vi "Test MFC ESF.vi"() -> ()   [LabVIEW 2015, in "Alicat Device.lvclass"]
uses:
  Alicat Device.lvclass
  Reusable/Session APIs/File Access/Config Data/Config Session.ctl
  Reusable/Session APIs/File Access/Config Data/Config Data.lvclass
  Reusable/Session APIs/Serial/Serial Session.lvclass
  <userlib>/_Session Fwk/Typedefs/Session Handle.ctl
  <userlib>/_Session Fwk/Session - Root.lvclass
  Reusable/Session Log/System Log.lvclass
  Reusable/Session Log/System Log.lvclass/System Log.ctl
  Reusable/Session APIs/File Access/Config Data/Config Data.lvclass/Config Data.ctl
  Reusable/Session APIs/Text Communication/Text Device Session.lvclass/Text Device Session.ctl
  Configurable Device/Configurable Device.lvclass/Configurable Device.ctl
  Alicat Device.lvclass/Alicat Device.ctl
  Data/M/M data.lvclass
  Data/Alicat Data.lvclass
  Data/M/M data.lvclass/M data.ctl
  Reusable/Session APIs/Text Communication/Write hSysLog.vi
  Configurable Device/Write Handle.vi
  Accessors/Write ID.vi
  Accessors/Write Session Handle.vi
  Data/M/Accessors/Read P.vi
  Data/M/Accessors/Read T.vi
  Reusable/Session APIs/File Access/Config Data/Accessors/Write Cfg Path.vi
  Reusable/Session Log/Accessors/Write Main Path.vi
  Reusable/Data/Read measTime.vi
panel:
  out "Numeric":u32
  out "Accessors:Data":sgl[][](array[numeric])
  out "Array 3":errorcluster[](array[cluster])
  out "Array 2":errorcluster[](array[cluster])
  in  "Stop":bool
  in  "Path":path=path "c:/aop/aop.ini"
  in  "Main Path":path=path "c:/aop/logs"
  in  "Array":string[](array[string])=["CRDS_Purge", "CRDS_Thermodenuded", "CRDS_Dry", "CRDS_Med_RH", "CRDS_High_RH"]
  out "Time":timestamp[](array[timestamp]) format="%<%H:%M:%S%2u>T"
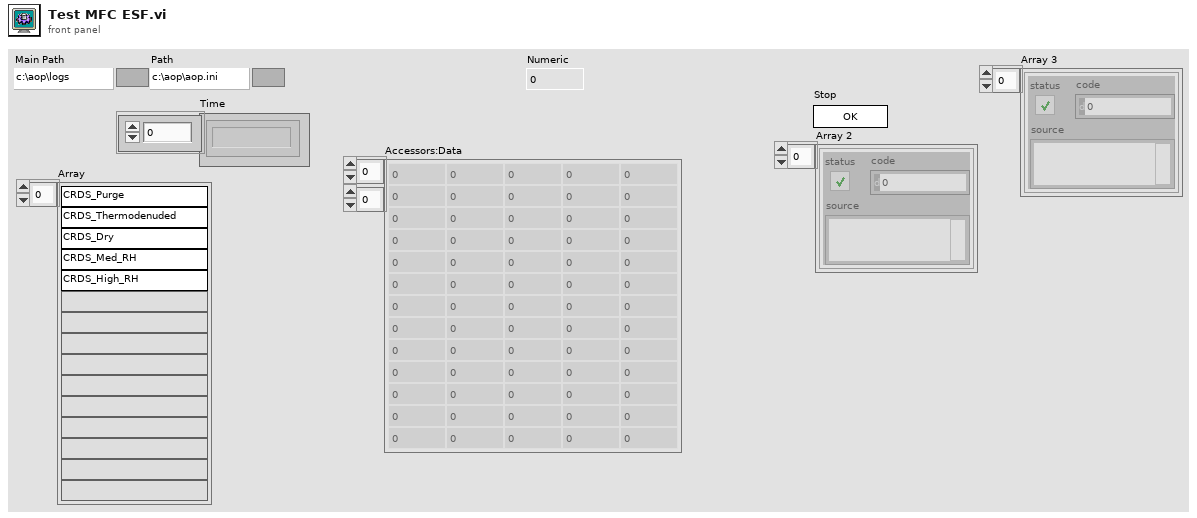
[diagram p1: front panel]
types:
  T1 = typedef "Session - Root.lvclass/Session Handle.ctl" = refnum<data-value>
  T2 = typedef "Config Data.lvclass/Config Session.ctl" = refnum<data-value>
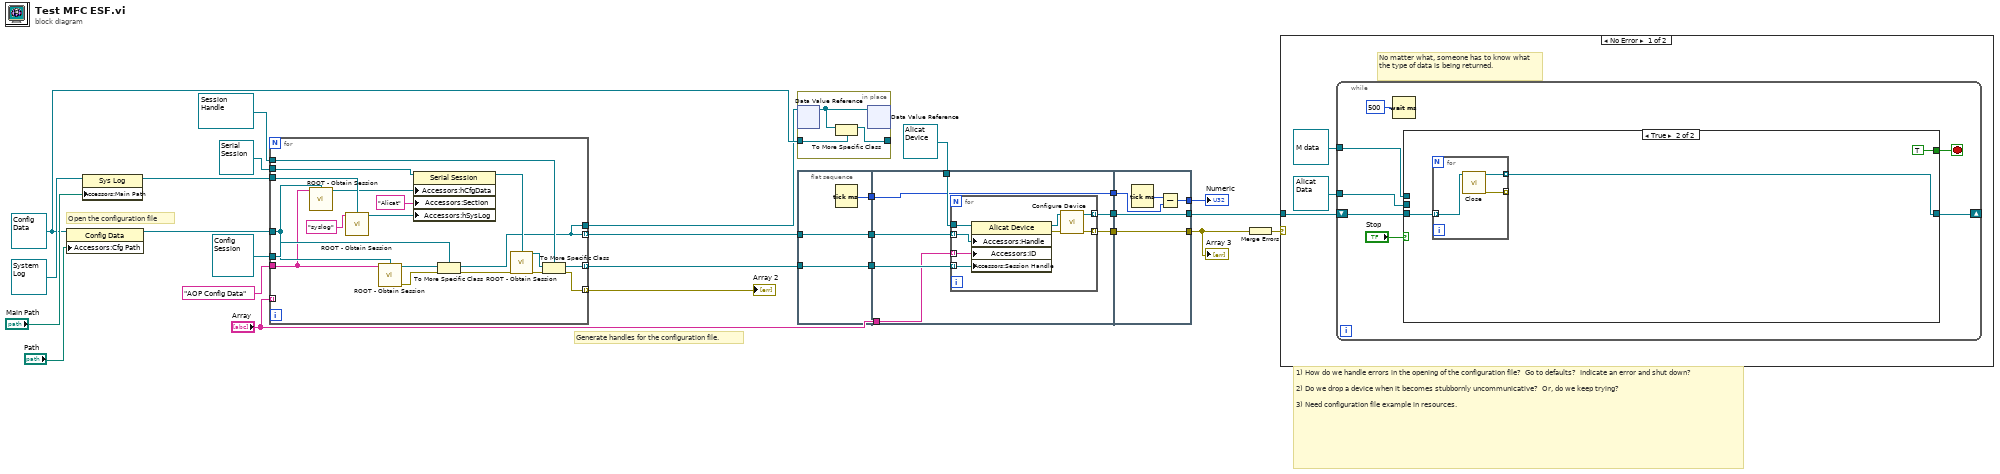
[diagram p0: block diagram]
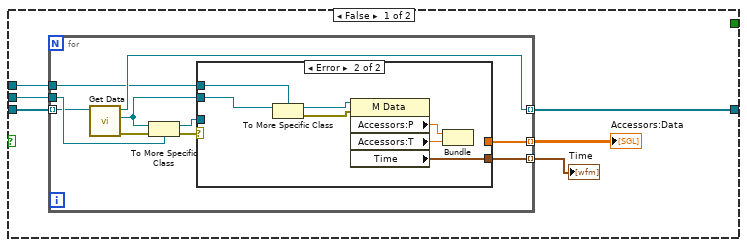
[diagram p2: hidden frame]
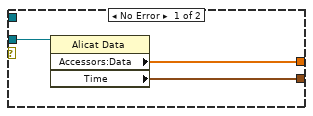
[diagram p3: hidden frame]
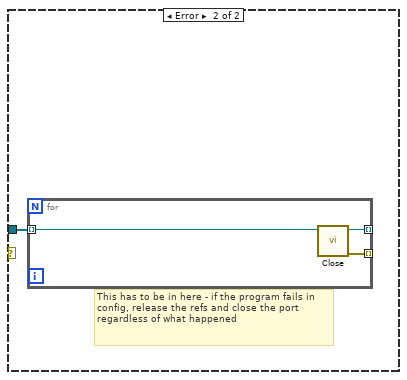
[diagram p4: hidden frame]
diagram:
  w9 = refnum<class "Config Data.lvclass"> refnum ("Config Data")
  # "1) How do we handle errors in the opening of the configuration file?  Go to defaults?  Indicate an error and shut down?\n\n2) Do we drop a device when it becomes stubbornly uncommunicative?  Or, do we keep trying?\n\n3) Need configuration file example in resources."
  # "Open the configuration file"
  # "Generate handles for the configuration file."
  n1 = property class="Config Data"(reference=w9, "Accessors:Cfg Path"="Path") -> (reference out=w12:refnum<class "Config Data.lvclass">)  [unwired: 1 in, 1 out]
  n2 = property class="Sys Log"(reference=refnum<class "System Log.lvclass"> refnum ("Sys Log"), "Accessors:Main Path"="Main Path") -> (reference out=w15:refnum<class "System Log.lvclass">)  [unwired: 1 in, 1 out]
  n3 = for {
    tunnel: T2 refnum ("Session Handle") -> [w45]
    tunnel: [w30] -> w10 mode=indexing
    tunnel: "AOP Config Data" ("Session Name ()") -> [w28]
    tunnel: refnum<class "Serial Session.lvclass"> refnum ("Serial Session") -> [w43]
    tunnel: T1 refnum ("Session Handle") -> [w39]
    tunnel: [w38] -> w18 mode=indexing
    tunnel: w15 -> [w37]
    tunnel: "Array" -> [_] mode=indexing
    tunnel: w12 -> [w29]
    tunnel: [w31] -> w11 mode=indexing
    tunnel: [w30] -> w8
    n4 = call <userlib>:"ROOT - Obtain Session.vi"("Session Name ()"=w28, "OBJ - Session"=w29) -> ("Session Handle"=w27:T1)  [unwired: 11 in, 2 out]
    n5 = call <userlib>:"ROOT - Obtain Session.vi"("Session Name ()"="syslog", "OBJ - Session"=w37) -> ("Session Handle"=w35:T1)  [unwired: 11 in, 2 out]
    n6 = call <userlib>:"ROOT - Obtain Session.vi"("Session Name ()"=w28, "OBJ - Session"=w29) -> ("Session Handle"=w34:T1, "error out"=w44:errorcluster)  [unwired: 11 in, 1 out]
    n7 = property class="Serial Session"(reference=w43, "Accessors:hCfgData"=w27, "Accessors:Section"="Alicat" ("Section"), "Accessors:hSysLog"=w35) -> (reference out=w42:refnum<class "Serial Session.lvclass">)  [unwired: 1 in, 1 out]
    n8 = To More Specific Class(target class=w45, reference=w34, error in=w44) -> (specific class reference=w30:T2, error out=w33:errorcluster)
    n9 = call <userlib>:"ROOT - Obtain Session.vi"("OBJ - Session"=w42, "error in (no error)"=w33) -> ("Session Handle"=w40:T1, "error out"=w32:errorcluster)  [unwired: 11 in, 1 out]
    n10 = To More Specific Class(target class=w39, reference=w40, error in=w32) -> (specific class reference=w38:T1, error out=w31:errorcluster)
  }
  "Array 2" <- w11
  n11 = in-place {
    in-place-border: w9 -> [w47]
    in-place-border: [w46] -> _
    n12 = in-place-dvr #1(w8) -> (w48:refnum<class "Config Data.lvclass">)  [unwired: 1 out]
    n13 = To More Specific Class(target class=w47, reference=w48) -> (specific class reference=w46:refnum<class "Config Data.lvclass">)  [unwired: 1 in, 1 out]
    n14 = in-place-dvr #1(w48) -> ()  [unwired: 2 out]
  }
  n15 = flat-sequence {
    tunnel: w10 -> [w50]
    tunnel: w18 -> [w51]
    tunnel: [w51] -> w5
    tunnel: [w50] -> w4
    tunnel: [w49] -> w2
    tunnel: refnum<class "Alicat Device.lvclass"> refnum ("Alicat Device in") -> [w56]
    tunnel: "Array" -> [w54]
    tunnel: [w58] -> w7
    tunnel: [w57] -> w6
    tunnel: w5 -> [w55]
    tunnel: w4 -> [w53]
    tunnel: [w52] -> w3
    tunnel: w2 -> [w52]
    tunnel: [w70] -> w24
    tunnel: [w71] -> w26
    tunnel: w7 -> [w71]
    tunnel: w6 -> [w70]
    tunnel: w3 -> [w68]
    tunnel: [w67] -> w1
    frame #0 {
      n16 = Tick Count (ms)() -> (millisecond timer value=w49:u32)
    }
    frame #1 {
      n17 = for {
        tunnel: w54 -> [w65] mode=indexing
        tunnel: [w61] -> w57 mode=indexing
        tunnel: [w60] -> w58 mode=indexing
        tunnel: w56 -> [w66]
        tunnel: w53 -> [w64] mode=indexing
        tunnel: w55 -> [w59] mode=indexing
        n18 = property class="Alicat Device"(reference=w66, "Accessors:Handle"=w64, "Accessors:ID"=w65, "Accessors:Session Handle"=w59) -> (reference out=w62:refnum<class "Alicat Device.lvclass">, error out=w63:errorcluster)  [unwired: 1 in]
        n19 = call-dynamic "Configure Device.vi"("error in"=w63, "Alicat Device in"=w62) -> ("error out"=w60:errorcluster, "Alicat Device out"=w61:refnum<class "Alicat Device.lvclass">)  [unwired: 8 in]
      }
    }
    frame #2 {
      n20 = Tick Count (ms)() -> (millisecond timer value=w69:u32)
      n21 = Subtract(x=w69, y=w68) -> (x-y=w67:u32)
    }
  }
  n22 = Merge Errors(w26) -> (w25:errorcluster)
  n23 = case shown="No Error" w25 {
    tunnel: w24 -> [w74 w114]
    frame No Error {
      # "No matter what, someone has to know what the type of data is being returned."
      n24 = while {
        shift-right: [w80] -> _
        shift-left: w74 -> [w81]
        tunnel: refnum<class "Alicat Data.lvclass"> refnum ("Alicat Data") -> [w79]
        tunnel: refnum<class "M data.lvclass"> refnum ("M Data") -> [w78]
        stop <- w76 stop-if-true
        n25 = Wait (ms)(milliseconds to wait=500) -> ()  [unwired: 1 out]
        n26 = case shown="True" "Stop" {
          tunnel: w81 -> [w87 w110]
          tunnel: [w86 w109] -> w80
          tunnel: w79 -> [w85 _]
          tunnel: w78 -> [w84 _]
          tunnel: [_ TRUE] -> w76
          frame False {
            n27 = for {
              tunnel: [w97] -> w86 mode=indexing
              tunnel: w85 -> [w95]
              tunnel: w87 -> [w93] mode=indexing
              tunnel: [w92] -> w83 mode=indexing
              tunnel: w84 -> [w90]
              tunnel: [w88] -> w82 mode=indexing
              n28 = call-dynamic "Get Data.vi"("Cfg Dev in"=w93) -> ("error out"=w96:errorcluster, "DataOut"=w89:refnum<class "Data.lvclass">, "Cfg Dev out"=w97:refnum<class "Alicat Device.lvclass">)  [unwired: 8 in]
              n29 = To More Specific Class(target class=w95, reference=w89, error in=w96) -> (specific class reference=w94:refnum<class "Alicat Data.lvclass">, error out=w91:errorcluster)
              n30 = case shown="Error" w91 {
                tunnel: w94 -> [w100 _]
                tunnel: [w99 w103] -> w92
                tunnel: w89 -> [_ w107]
                tunnel: w90 -> [_ w106]
                tunnel: [w98 _] -> w88
                frame No Error {
                  n31 = property class="Alicat Data"(reference=w100) -> ("Accessors:Data"=w98:sgl[], "Time"=w99:timestamp)  [unwired: 1 in, 2 out]
                }
                frame Error {
                  n32 = To More Specific Class(target class=w106, reference=w107) -> (specific class reference=w104:refnum<class "M data.lvclass">, error out=w105:errorcluster)  [unwired: 1 in]
                  n33 = property class="M Data"(reference=w104, error in=w105) -> ("Accessors:P"=w102:sgl, "Accessors:T"=w101:sgl, "Time"=w103:timestamp)  [unwired: 2 out]
                  n34 = Bundle("Accessors:P"=w102, "Accessors:T"=w101) -> ()  [unwired: 1 in, 1 out]
                }
              }
            }
            "Time" <- w83
            "Accessors:Data" <- w82
          }
          frame True {
            n35 = for {
              tunnel: [w112] -> w109 mode=indexing
              tunnel: [w111] -> _ mode=indexing
              tunnel: w110 -> [w113] mode=indexing
              n36 = call-dynamic "Close.vi"("Cfg Dev in"=w113) -> ("error out"=w111:errorcluster, "Cfg Dev out"=w112:refnum<class "Alicat Device.lvclass">)  [unwired: 9 in]
            }
          }
        }
      }
    }
    frame Error {
      # "This has to be in here - if the program fails in config, release the refs and close the port regardless of what happened"
      n37 = for {
        tunnel: [w116] -> _ mode=indexing
        tunnel: [w115] -> _ mode=indexing
        tunnel: w114 -> [w117] mode=indexing
        n38 = call-dynamic "Close.vi"("Cfg Dev in"=w117) -> ("error out"=w115:errorcluster, "Cfg Dev out"=w116:refnum<class "Alicat Device.lvclass">)  [unwired: 9 in]
      }
    }
  }
  "Array 3" <- w26
  "Numeric" <- w1
